vi "Ev Save.vi"(8 "error in (no error)":errorcluster, 11 "Configuration Window in":refnum<class "Configuration Window.lvclass">) -> (0 "error out":errorcluster, 3 "Configuration Window out":refnum<class "Configuration Window.lvclass">)   [LabVIEW 2018, in "Configuration Window.lvlib" / "Configuration Window.lvclass"]
uses:
  Configuration Window.lvclass
  C:/Program Files (x86)/National Instruments/LabVIEW 2018/vi.lib/ActorFramework/Actor/Actor.lvclass
  <vilib>/ActorFramework/Actor/Actor.lvclass/Actor.ctl
  <vilib>/ActorFramework/Message Enqueuer/Message Enqueuer.lvclass/Message Enqueuer.ctl
  <vilib>/ActorFramework/Message Enqueuer/Init from Existing Queue.vi
  <vilib>/ActorFramework/Message Enqueuer/Enqueue.vi
  <vilib>/ActorFramework/Stop Msg/Stop Msg.lvclass
  C:/Program Files (x86)/National Instruments/LabVIEW 2018/vi.lib/ActorFramework/Message/Message.lvclass
  <vilib>/ActorFramework/Message Priority Queue/Priority Enqueue.vi
  <vilib>/ActorFramework/Message Enqueuer/Message Enqueuer.lvclass
  <vilib>/ActorFramework/Actor/Actor.lvclass
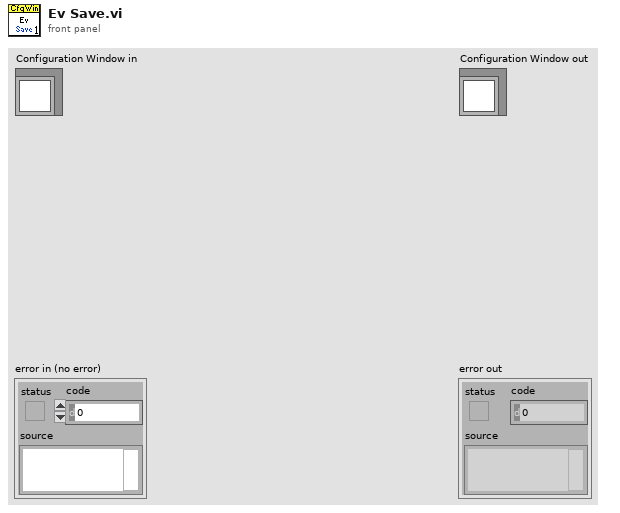
[diagram p1: front panel]
types:
  T1 = typedef "Main Panel.lvlib/Main Panel.lvclass/Const Configuration.ctl" = cluster{"Language":cluster{"Name":string}, "Path Config":T2, "Image Viewer Config":T3}
  T2 = typedef "Main Panel.lvlib/Main Panel.lvclass/Const Path Setting.ctl" = cluster{"Data Folder Path":path, "PNG Folder Path":path}
  T3 = typedef "Main Panel.lvlib/Main Panel.lvclass/Const Image Viewer Setting.ctl" = cluster{"Center Point":cluster{"Size":i32, "Color":u32, "Show?":bool}, "bp Point":cluster{"Size":i32, "Color":u32, "Show?":bool}, "w Point":cluster{"Size":i32, "Color":u32, "Show?":bool}, "b Box":cluster{"Fill Color":u32, "Border Color":u32, "Show?":bool}, "i Box":cluster{"Fill Color":u32, "Border Color":u32, "Show?":bool}, "o Point":cluster{"Size":i32, "Color":u32, "Show?":bool}, "c Point":cluster{"Size":i32, "Color":u32, "Show?":bool}}
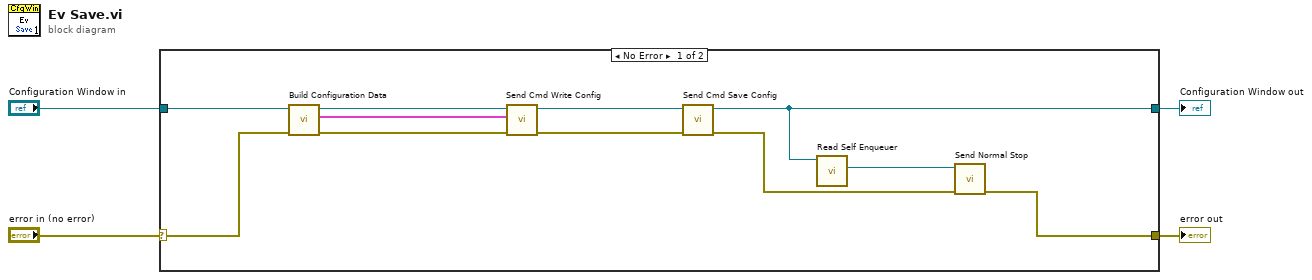
[diagram p0: block diagram]
diagram:
  n1 = case shown="No Error" "error in (no error)" {
    selector: "error in (no error)" -> [w9 w17]
    tunnel: [w14 w17] -> w3
    tunnel: [w7 w16] -> w1
    tunnel: "Configuration Window in" -> [w10 w16]
    frame No Error {
      n2 = call "Build Configuration Data.vi"("error in (no error)"=w9, "Configuration Window in"=w10) -> ("error out"=w12:errorcluster, "Configuration"=w11:T1, "Configuration Window out"=w13:refnum<class "Configuration Window.lvclass">)  [unwired: 7 in]
      n3 = call "Send Cmd Write Config.vi"("error in (no error)"=w12, "Configuration"=w11, "Configuration Window in"=w13) -> ("error out"=w6:errorcluster, "Configuration Window out"=w8:refnum<class "Configuration Window.lvclass">)  [unwired: 7 in]
      n4 = call "Send Cmd Save Config.vi"("error in (no error)"=w6, "Configuration Window in"=w8) -> ("error out"=w5:errorcluster, "Configuration Window out"=w7:refnum<class "Configuration Window.lvclass">)  [unwired: 8 in]
      n5 = call <vilib>:"Read Self Enqueuer.vi"("Actor"=w7) -> ("Self Enqueuer"=w15:refnum<class "Message Enqueuer.lvclass">)  [unwired: 10 in]
      n6 = call <vilib>:"Send Normal Stop.vi"("error in (no error)"=w5, "Message Enqueuer"=w15) -> ("error out"=w14:errorcluster)  [unwired: 9 in]
    }
    frame Error {
    }
  }
  "error out" <- w3
  "Configuration Window out" <- w1
